vi "Read status.vi"(1 "Port":T2={"P type"=0, "reference"="", " Terminator "="\r\n", "Timeout"=300} {"Timeout" step=10; "P type" items=["none", "RS-232C"]}, 3 "error in (no error)":errorcluster, 5 "Controller #":string) -> (6 "Status":T1(ring), 7 "Error?":bool, 9 "status array":bool[](array[boolean]), 10 "error out":errorcluster)   [LabVIEW 2013]
panel:
  # "Read status"
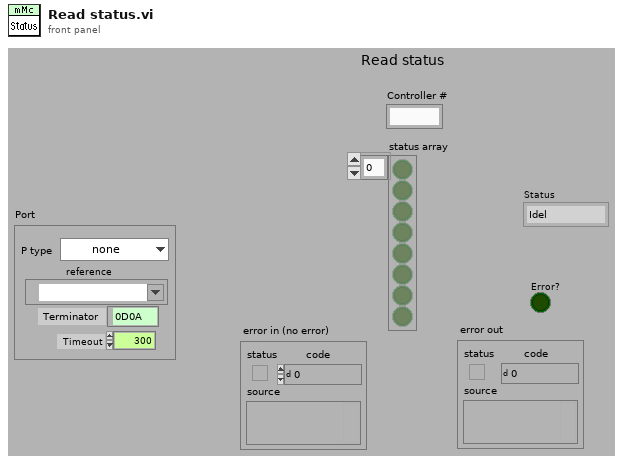
[diagram p1: front panel]
types:
  T1 = enum16{"Idel", "Moving", "Accelerating", "Decelerating", "L- (neg limit)", "L+ (pos limit)", "Homed", "Unknown"}
  T2 = cluster{"P type":u16, "reference":refnum<visa-resource-name>, " Terminator ":string, "Timeout":i32}
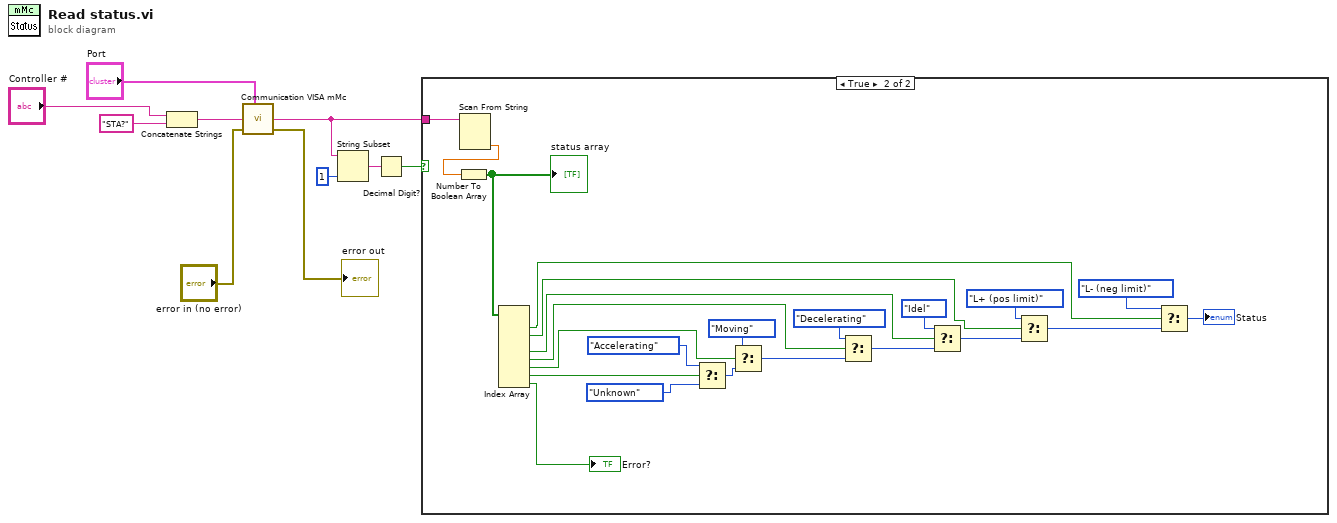
[diagram p0: block diagram]
diagram:
  n1 = Concatenate Strings("Controller #", "STA?") -> (w6:string)
  n2 = call "Communication VISA mMc.vi"("Port"="Port", "Command"=w6, "error in (no error)"="error in (no error)") -> ("Return"=w1:string, "error out"=→"error out":errorcluster)  [unwired: 3 in, 2 out]
  n3 = String Subset(string=w1, length (rest)=1 ("length (rest)")) -> (substring=w3:string)  [unwired: 1 in]
  n4 = Decimal Digit?(1:w3) -> (0:w2:bool)
  n5 = case shown="True" w2 {
    tunnel: w1 -> [_ w33]
    frame False {
    }
    frame True {
      n6 = Scan From String(input string=w33) -> (output 1=w32:dbl)  [unwired: 4 in, 3 out]
      n7 = Number To Boolean Array(number=w32) -> (Boolean array=w31:bool[])
      "status array" <- w31
      n8 = Index Array(array=w31) -> (element #1=w13:bool, element #2=w14:bool, element #4=w15:bool, element #5=w16:bool, element #6=w17:bool, element #7=w18:bool, element #8=→"Error?":bool)  [unwired: 8 in, 1 out]
      n9 = Select(t=T1."Accelerating" ("Settings.Motor status"), s=w18, f=T1."Unknown" ("Settings.Motor status")) -> (s? t:f=w28:T1)
      n10 = Select(t=T1."Moving" ("Settings.Motor status"), s=w17, f=w28) -> (s? t:f=w26:T1)
      n11 = Select(t=T1."Decelerating" ("Settings.Motor status"), s=w16, f=w26) -> (s? t:f=w24:T1)
      n12 = Select(t=T1."Idel" ("Settings.Motor status"), s=w15, f=w24) -> (s? t:f=w21:T1)
      n13 = Select(t=T1."L+ (pos limit)" ("Settings.Motor status"), s=w14, f=w21) -> (s? t:f=w20:T1)
      n14 = Select(t=T1."L- (neg limit)" ("Settings.Motor status"), s=w13, f=w20) -> (s? t:f=→"Status":T1)
    }
  }
